vi "Station.Buttons.Check.vi"(8 "error in":errorcluster) -> (0 "error out":errorcluster, 1 "Buttons array":bool[](array[boolean]), 2 "Buttons":T1)   [LabVIEW 2016]
uses:
  Station.Buttons.ctl
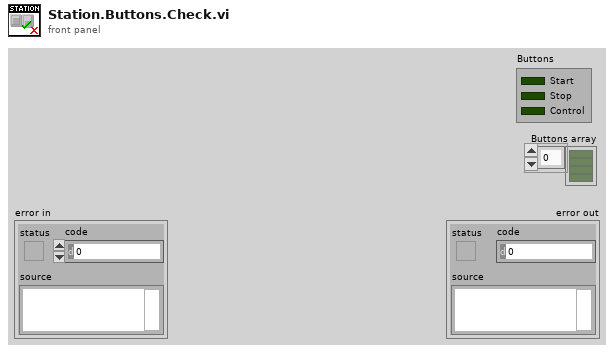
[diagram p1: front panel]
types:
  T1 = typedef "Station.Buttons.ctl" = cluster{"Start":bool, "Stop":bool, "Control":bool}
  T2 = typedef "FestoCPX.Station.ButtonsState.ctl" = cluster{"Start":bool, "Stop":bool, "Control":bool}
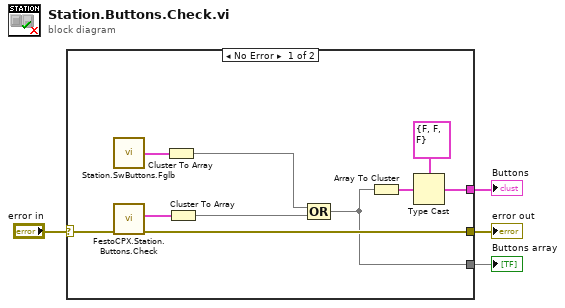
[diagram p0: block diagram]
diagram:
  n1 = case shown="No Error" "error in" {
    selector: "error in" -> [w9 w15]
    tunnel: [w8 w15] -> w4
    tunnel: [w11 _] -> w1
    tunnel: [w5 _] -> w2
    frame No Error {
      n2 = call "Station.SwButtons.Fglb.vi"() -> ("Buttons"=w10:T1)  [unwired: 2 in]
      n3 = call "FestoCPX.Station.Buttons.Check.vi"("error in"=w9) -> ("error out"=w8:errorcluster, "Buttons.State"=w7:T2)  [unwired: 9 in]
      n4 = Cluster To Array(cluster=w10) -> (array=w13:bool[])
      n5 = Cluster To Array(cluster=w7) -> (array=w6:bool[])
      n6 = Compound Arithmetic op=OR(w13, w6) -> (w5:bool[])
      n7 = Array To Cluster(array=w5) -> (cluster=w14:cluster{"[0]":bool, "[1]":bool, "[2]":bool})
      n8 = Type Cast(type=T1 {"Start"=FALSE, "Stop"=FALSE, "Control"=FALSE} ("Buttons"), x=w14) -> (*(type *) &x=w11:T1)
    }
    frame Error {
    }
  }
  "error out" <- w4
  "Buttons array" <- w2
  "Buttons" <- w1
